vi "LabVIEWArduino2.vi"() -> ()   [LabVIEW 2020]
uses:
  <vilib>/Instr/_visa.llb/VISA Configure Serial Port (Instr).vi
panel:
  out "match substring":string
  in  "termination char\n(0xA = '\\n' = LF)":u8=10 format="%.0x"
  out "Waveform Graph":dbl[](graph)
  in  "VISA resource name":refnum<visa-resource-name>="COM3"
  in  "data bits (8)":u16=8 min=5 max=8 step=1
  in  "stop bits (10: 1 bit)":u16(ring)=10 items=["1.0"=10, "1.5"=15, "2.0"=20]
  in  "flow control (0:none)":u16(ring) items=["None", "XON/XOFF", "RTS/CTS", "XON/XOFF & RTS/CTS", "DTR/DSR", "XON/XOFF & DTR/DSR"]
  in  "parity (0:none)":enum16{"None", "Odd", "Even", "Mark", "Space"}(ring)
  out "TempArray":dbl[](array[numeric]) caption="Temperature Array"
  out "CurTemp":dbl caption="Current Temperature\n(Celsius)"
  in  "stop":bool
  in  "LabVIEW Stop":bool
  out "LabVIEW Echo":string
  in  "Emergency Stop!":bool
  in  "Decellerate":bool
  in  "Motor Control Duino":refnum<visa-resource-name>
  in  "Accelerate":bool
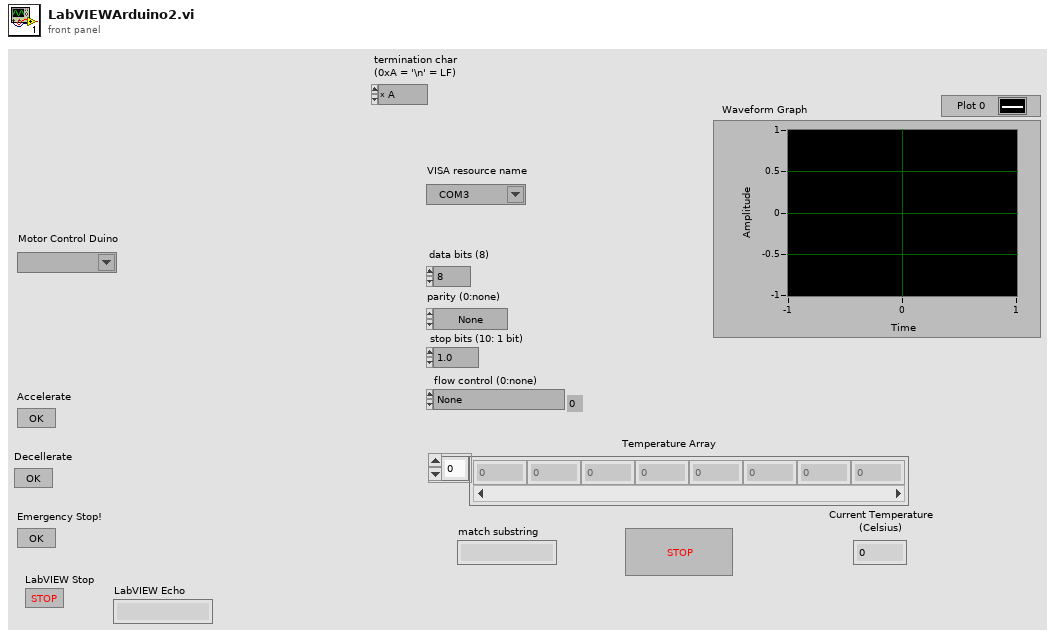
[diagram p1: front panel]
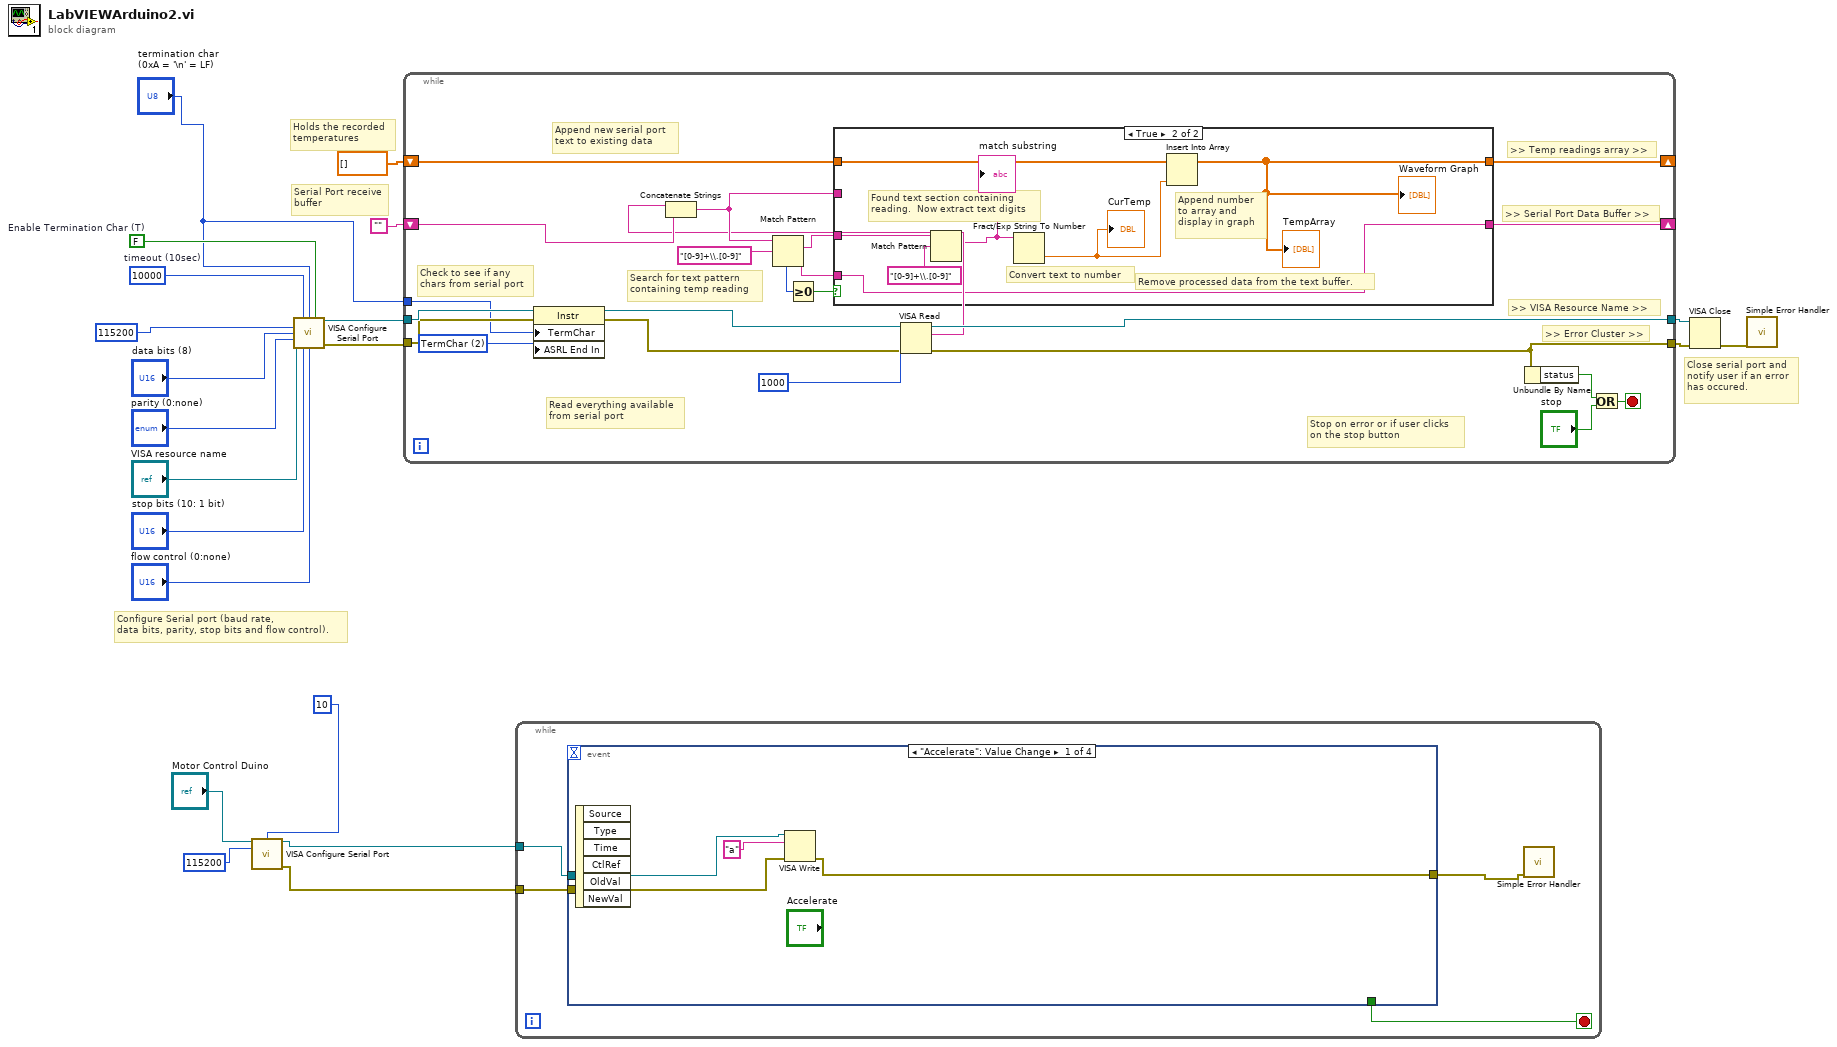
[diagram p0: block diagram]
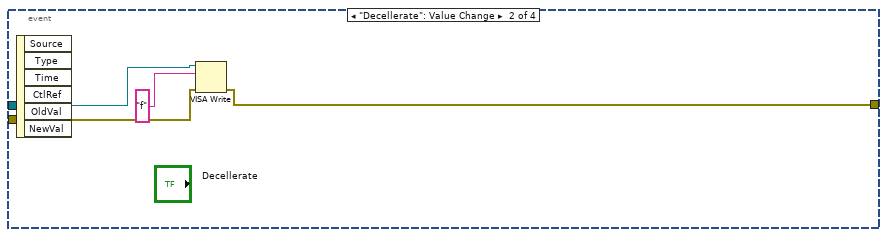
[diagram p3: hidden frame]
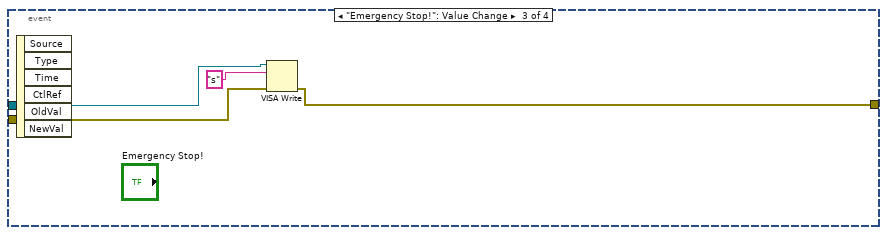
[diagram p4: hidden frame]
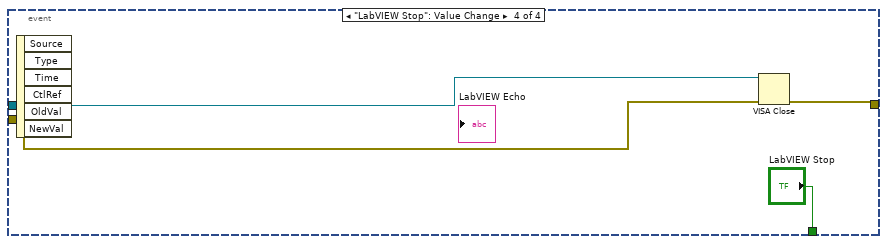
[diagram p5: hidden frame]
diagram:
  w15 = FALSE  # Enable Termination Char (T)
  w16 = u32 10000  # timeout (10sec)
  # "Close serial port and\nnotify user if an error\nhas occured."
  # "Serial Port receive\nbuffer"
  # "Holds the recorded\ntemperatures"
  # "Configure Serial port (baud rate,\ndata bits, parity, stop bits and flow control)."
  n1 = call-poly "VISA Configure Serial Port"("VISA resource name"="Motor Control Duino", "termination char\n(0xA = '\\n' = LF)"=u8 10 ("termination char\n(0xA = '\\n' = LF)"), "baud rate (9600)"=u32 115200) -> ("VISA resource name out"=w3:refnum<visa-resource-name>, "error out"=w2:errorcluster)  [unwired: 11 in]
  n2 = call-poly "VISA Configure Serial Port"("VISA resource name"="VISA resource name", "timeout (10sec)"=w16, "termination char\n(0xA = '\\n' = LF)"="termination char\n(0xA = '\\n' = LF)", "Enable Termination\nChar (T)"=w15, "baud rate (9600)"=u32 115200, "data bits (8)"="data bits (8)", "parity (0:none)"="parity (0:none)", "stop bits (10: 1 bit)"="stop bits (10: 1 bit)", "flow control (0:none)"="flow control (0:none)") -> ("VISA resource name out"=w5:refnum<visa-resource-name>, "error out"=w4:errorcluster)  [unwired: 5 in]
  n3 = while {
    tunnel: [w42] -> w19
    tunnel: [w44] -> w18
    shift-right: [w36] -> _
    shift-left: "" -> [w43]
    tunnel: w5 -> [w27]
    tunnel: w4 -> [w26]
    shift-right: [w38] -> _
    shift-left: dbl[] [] -> [w37]
    tunnel: "termination char\n(0xA = '\\n' = LF)" -> [w23]
    stop <- w41 stop-if-true
    w22 = u16 2 items=["None", "Last Bit", "TermChar"] ("Serial Settings:End Mode for Reads")
    # "Search for text pattern\ncontaining temp reading"
    # "Append new serial port\ntext to existing data"
    # "Read everything available\nfrom serial port"
    # "Stop on error or if user clicks \non the stop button"
    # ">> Error Cluster >>"
    # ">> VISA Resource Name >>"
    # ">> Temp readings array >>"
    # ">> Serial Port Data Buffer >>"
    # "Check to see if any\nchars from serial port"
    n4 = property class="Instr"(reference=w27, error in=w26, "TermChar"=w23, "ASRL End In"=w22) -> (reference out=w25:refnum<visa-resource-name>, error out=w24:errorcluster)
    n5 = VISA Read(VISA resource name=w25, byte count=u32 1000, error in (no error)=w24) -> (VISA resource name out=w44:refnum<visa-resource-name>, read buffer=w29:string, error out=w42:errorcluster)  [unwired: 1 out]
    n6 = Concatenate Strings(w29, w43) -> (w30:string)
    n7 = Match Pattern(string=w30, regular expression="[0-9]+\\.[0-9]") -> (match substring=w32:string, after substring=w31:string, offset past match=w34:i32)  [unwired: 1 in, 1 out]
    n8 = Greater Or Equal To 0?(x=w34) -> (x >= 0?=w33:bool)
    n9 = case shown="True" w33 {
      tunnel: w32 -> [_ w52]
      tunnel: w31 -> [_ w53]
      tunnel: w30 -> [w46 _]
      tunnel: [w46 w53] -> w36
      tunnel: [w45 w47] -> w38
      tunnel: w37 -> [w45 w50]
      frame False {
        # "Did not find text pattern in the buffer.  Try again in the next loop after new data \nhas been received."
      }
      frame True {
        # "Remove processed data from the text buffer."
        # "Append number\nto array and\ndisplay in graph"
        # "Convert text to number"
        # "Found text section containing \nreading.  Now extract text digits"
        n10 = Match Pattern(string=w52, regular expression="[0-9]+\\.[0-9]") -> (match substring=w51:string)  [unwired: 1 in, 3 out]
        "match substring" <- w51
        n11 = Fract/Exp String To Number(string=w51) -> (number=w48:dbl)  [unwired: 3 in, 1 out]
        "CurTemp" <- w48
        n12 = Insert Into Array(array=w50, new element=w48) -> (w47:dbl[])  [unwired: 1 in]
        "TempArray" <- w47
        "Waveform Graph" <- w47
      }
    }
    n13 = Unbundle By Name(w42) -> ("status"=w40:bool)
    n14 = Or(x=w40, y="stop") -> (x .or. y?=w41:bool)
  }
  n15 = while {
    tunnel: w3 -> [w57]
    tunnel: w2 -> [w56]
    stop <- w54 stop-if-true
    n16 = event shown="[0] \"Accelerate\": Value Change" {
      selector: _ -> [_ _ _ _]
      dyn-events: _ -> [_ _ _ _]
      timeout: _ -> [_ _ _ _]
      tunnel: [w61 w65 w69 w73] -> w55
      tunnel: w57 -> [w60 w63 w67 w72]
      tunnel: w56 -> [w59 w62 w66 w71]
      tunnel: [_ _ _ "LabVIEW Stop"] -> w54
      event "Accelerate": Value Change {
        n17 = event-data() -> ()  [unwired: 1 in, 6 out]
        n18 = VISA Write(VISA resource name=w60, write buffer="a", error in (no error)=w59) -> (error out=w61:errorcluster)  [unwired: 2 out]
      }
      event "Decellerate": Value Change {
        n19 = event-data() -> ()  [unwired: 1 in, 6 out]
        n20 = VISA Write(VISA resource name=w63, write buffer="f", error in (no error)=w62) -> (error out=w65:errorcluster)  [unwired: 2 out]
      }
      event "Emergency Stop!": Value Change {
        n21 = event-data() -> ()  [unwired: 1 in, 6 out]
        n22 = VISA Write(VISA resource name=w67, write buffer="s", error in (no error)=w66) -> (error out=w69:errorcluster)  [unwired: 2 out]
      }
      event "LabVIEW Stop": Value Change {
        n23 = event-data() -> ()  [unwired: 1 in, 6 out]
        n24 = VISA Close(VISA resource name=w72, error in (no error)=w71) -> (error out=w73:errorcluster)
      }
    }
    n25 = call <vilib>:"Simple Error Handler.vi"("error in (no error)"=w55) -> ()  [unwired: 4 in, 5 out]
  }
  n26 = VISA Close(VISA resource name=w18, error in (no error)=w19) -> (error out=w17:errorcluster)
  n27 = call <vilib>:"Simple Error Handler.vi"("error in (no error)"=w17) -> ()  [unwired: 4 in, 5 out]
